vi "solar Msg Other (Broadcast).vi"(8 "error in (no error)":errorcluster, 9 "TLM_DATA":variant, 10 "TLM":string, 11 "solar in":refnum<class "solar.lvclass">) -> (0 "error out":errorcluster, 3 "solar out":refnum<class "solar.lvclass">)   [LabVIEW 2018]
doc: "This broadcasts the message to all subscribed queues and user events. The messages broadcast prefix this target's name as 'TARGET:TLM'"
uses:
  solar.lvclass
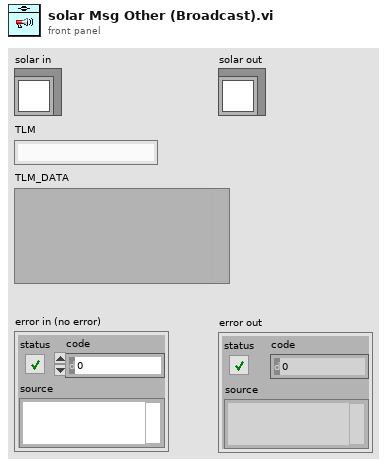
[diagram p1: front panel]
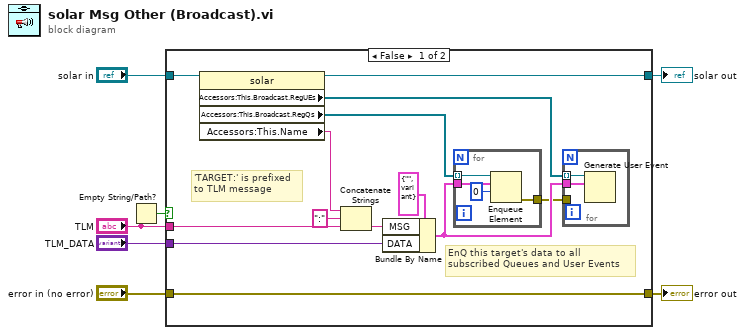
[diagram p0: block diagram]
diagram:
  n1 = Empty String/Path?(string/path="TLM") -> (empty?=w1:bool)
  n2 = case shown="False" w1 {
    tunnel: "solar in" -> [w20 w28]
    tunnel: [w19 w28] -> w6
    tunnel: "TLM_DATA" -> [w12 _]
    tunnel: "error in (no error)" -> [w14 w27]
    tunnel: "TLM" -> [w15 _]
    tunnel: [w14 w27] -> w2
    frame False {
      # "'TARGET:' is prefixed\nto TLM message"
      # "EnQ this target's data to all\nsubscribed Queues and User Events"
      n3 = property class="solar"(reference=w20) -> (reference out=w19:refnum<class "solar.lvclass">, "Accessors:This.Broadcast.RegUEs"=w17:refnum<user-event>[], "Accessors:This.Broadcast.RegQs"=w18:refnum<queue>[], "Accessors:This.Name"=w10:string)  [unwired: 1 in, 1 out]
      n4 = Concatenate Strings(w10, ":" ("string"), w15) -> (w11:string)
      n5 = Bundle By Name(cluster=cluster{"MSG":string, "DATA":variant} {"MSG"="", "DATA"=variant} ("MSG"), "MSG"=w11, "DATA"=w12) -> (w16:cluster{"MSG":string, "DATA":variant})
      n6 = for {
        tunnel: w18 -> [w23] mode=indexing
        tunnel: w16 -> [w22]
        tunnel: [w21] -> w8
        n7 = Enqueue Element(queue=w23, element=w22, timeout in ms (-1)=0) -> (error out=w21:errorcluster)  [unwired: 1 in, 2 out]
      }
      n8 = for {
        tunnel: w17 -> [w26] mode=indexing
        tunnel: w16 -> [w25]
        tunnel: w8 -> [_]
        n9 = Generate User Event(user event=w26, event data cluster=w25) -> ()  [unwired: 2 in, 2 out]
      }
    }
    frame True {
    }
  }
  "error out" <- w2
  "solar out" <- w6
